vi "TCPServiceInit.vi"(2 "Type":string="baxter_core_msgs/ListCameras", 3 "topic":string, 4 "callerID":string) -> (1 "TCP ROS Reply":string)   [LabVIEW 2015]
doc: "Initiates a service client"
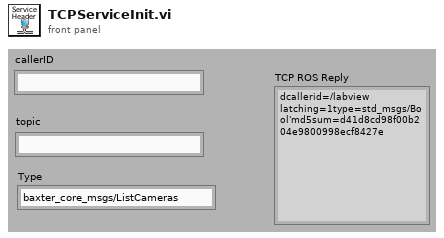
[diagram p1: front panel]
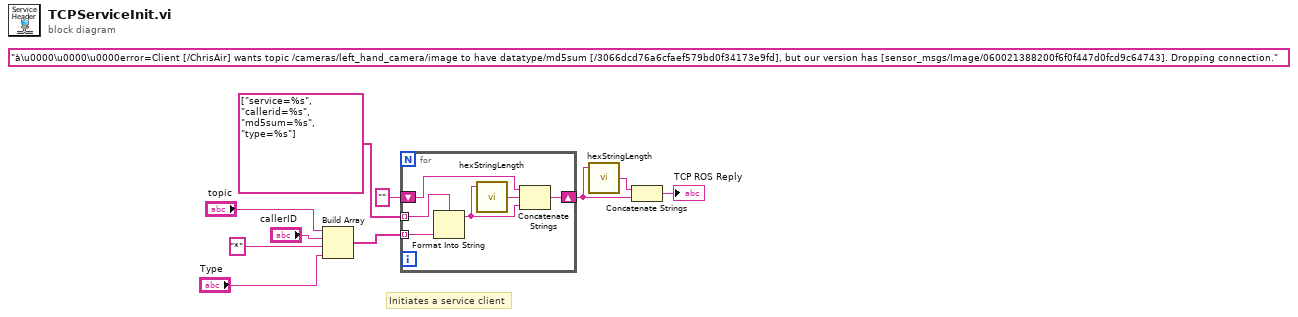
[diagram p0: block diagram]
diagram:
  (unwired) "à\u0000\u0000\u0000error=Client [/ChrisAir] wants topic /cameras/left_hand_camera/image to have datatype/md5sum [/3066dcd76a6cfaef579bd0f34173e9fd], but our version has [sensor_msgs/Image/060021388200f6f0f447d0fcd9c64743]. Dropping connection." ("Second")
  # "Initiates a service client"
  n1 = Build Array("topic", "callerID", "*", "Type") -> (w5:string[])
  n2 = for {
    tunnel: w5 -> [w15] mode=indexing
    tunnel: string[] ["service=%s", "callerid=%s", "md5sum=%s", "type=%s"] -> [w16] mode=indexing
    shift-right: [w11] -> w10
    shift-left: "" -> [w12]
    n3 = Format Into String(format string=w16, w15) -> (resulting string=w13:string)  [unwired: 2 in, 1 out]
    n4 = call "hexStringLength.vi"("String"=w13) -> ("String hex length"=w14:string)  [unwired: 2 in]
    n5 = Concatenate Strings(w12, w14, w13) -> (w11:string)
  }
  n6 = call "hexStringLength.vi"("String"=w10) -> ("String hex length"=w7:string)  [unwired: 2 in]
  n7 = Concatenate Strings(w7, w10) -> (→"TCP ROS Reply":string)
